vi "PC104_interface.vi"() -> ()   [LabVIEW 2016]
uses:
  Type_Defs/Digital_Out.ctl
  Type_Defs/Digital_In_1.ctl
  <vilib>/httpClient/ClientHandle.ctl
  Type_Defs/Analog_In.ctl
  msg7171_linux.llb/send single message.vi
  msg7171_linux.llb/send multiple messages.vi
  <vilib>/httpClient/POSTBuffer.vi
  <vilib>/httpClient/LabVIEWHTTPClient.lvlib
panel:
  out "GetAIO json":string
  out "GetDIO json":string
  in  "Get AIO":bool=TRUE
  in  "IR Lamps DutyCycle":dbl[][](array[numeric])
  in  "LN2 Platen":u16(slide) max=4095 step=1 scale=0.0..4095.0
  in  "LN2 Shroud":u16(slide) max=4095 step=1 scale=0.0..4095.0
  out "Digi_In_1":T1
  in  "Digi_Out":T2
  in  "Get DIO":bool=TRUE
  in  "exit":bool
  # "1"
  # "15"
  # "2"
  # "16"
  # "2               4                6                8                10              12              14              16"
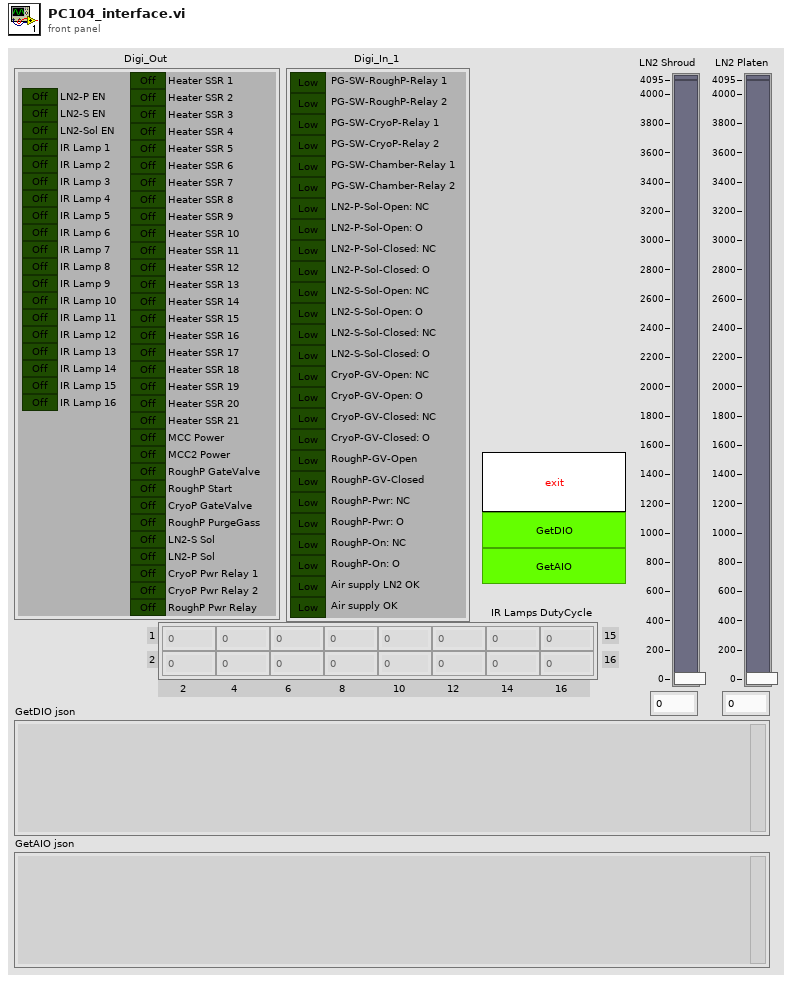
[diagram p1: front panel]
types:
  T1 = typedef "Digital_In_1.ctl" = cluster{"PG-SW-RoughP-Relay 1":bool, "PG-SW-RoughP-Relay 2":bool, "PG-SW-CryoP-Relay 1":bool, "PG-SW-CryoP-Relay 2":bool, "PG-SW-Chamber-Relay 1":bool, "PG-SW-Chamber-Relay 2":bool, "LN2-P-Sol-Open: NC":bool, "LN2-P-Sol-Open: O":bool, "LN2-P-Sol-Closed: NC":bool, "LN2-P-Sol-Closed: O":bool, "LN2-S-Sol-Open: NC":bool, "LN2-S-Sol-Open: O":bool, "LN2-S-Sol-Closed: NC":bool, "LN2-S-Sol-Closed: O":bool, "CryoP-GV-Open: NC":bool, "CryoP-GV-Open: O":bool, "CryoP-GV-Closed: NC":bool, "CryoP-GV-Closed: O":bool, "RoughP-GV-Open":bool, "RoughP-GV-Closed":bool, "RoughP-Pwr: NC":bool, "RoughP-Pwr: O":bool, "RoughP-On: NC":bool, "RoughP-On: O":bool, "Air supply LN2 OK":bool, "Air supply OK":bool}
  T2 = typedef "Digital_Out.ctl" = cluster{"LN2-P EN":bool, "LN2-S EN":bool, "LN2-Sol EN":bool, "IR Lamp 1":bool, "IR Lamp 2":bool, "IR Lamp 3":bool, "IR Lamp 4":bool, "IR Lamp 5":bool, "IR Lamp 6":bool, "IR Lamp 7":bool, "IR Lamp 8":bool, "IR Lamp 9":bool, "IR Lamp 10":bool, "IR Lamp 11":bool, "IR Lamp 12":bool, "IR Lamp 13":bool, "IR Lamp 14":bool, "IR Lamp 15":bool, "IR Lamp 16":bool, "Heater SSR 1":bool, "Heater SSR 2":bool, "Heater SSR 3":bool, "Heater SSR 4":bool, "Heater SSR 5":bool, "Heater SSR 6":bool, "Heater SSR 7":bool, "Heater SSR 8":bool, "Heater SSR 9":bool, "Heater SSR 10":bool, "Heater SSR 11":bool, "Heater SSR 12":bool, "Heater SSR 13":bool, "Heater SSR 14":bool, "Heater SSR 15":bool, "Heater SSR 16":bool, "Heater SSR 17":bool, "Heater SSR 18":bool, "Heater SSR 19":bool, "Heater SSR 20":bool, "Heater SSR 21":bool, "MCC Power":bool, "MCC2 Power":bool, "RoughP GateValve":bool, "RoughP Start":bool, "CryoP GateValve":bool, "RoughP PurgeGass":bool, "LN2-S Sol":bool, "LN2-P Sol":bool, "CryoP Pwr Relay 1":bool, "CryoP Pwr Relay 2":bool, "RoughP Pwr Relay":bool}
  T3 = typedef "LabVIEWHTTPClient.lvlib/ClientHandle.ctl" = refnum<k1>
  T4 = cluster{"go":bool, "Http session":T3, "URL prefex":string}
  T5 = typedef "Analog_In.ctl" = cluster{"Cabinet Temp 1":u16, "Cabinet Temp 2":u16, "Cabinet Temp 3":u16, "fs Front Door 1":u16, "fs Front Door 2":u16, "fs Front Door 3":u16, "fs Back Door 1":u16, "fs Back Door 2":u16, "fs Back Door 3":u16, "Rough Pump Temp":u16, "pg Chamber":u16, "pg Cryo Pump":u16, "pg Rough Pump":u16, "LN2 platen":u16, "LN2 shroud":u16}
  T6 = cluster{"out":cluster{"LN2 Platen":u16, "LN2 Shroud":u16}, "in":T5}
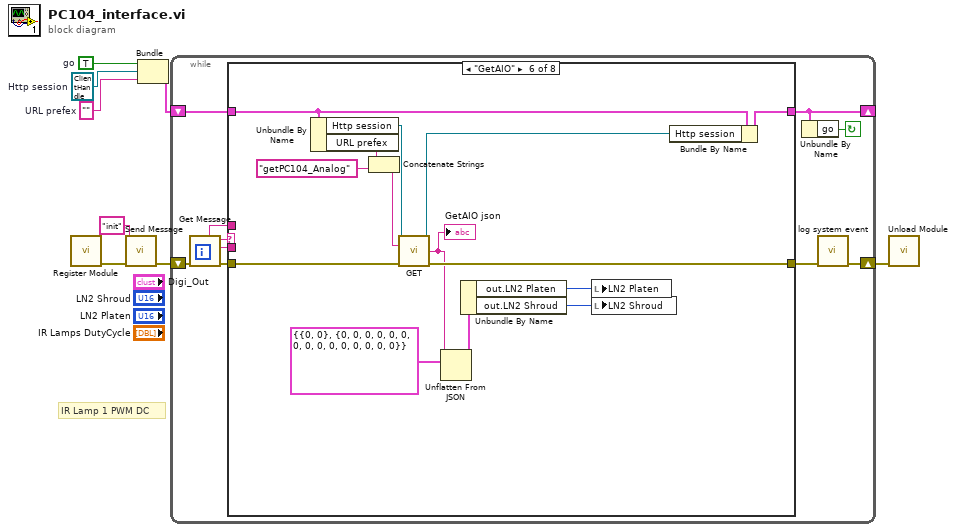
[diagram p0: block diagram]
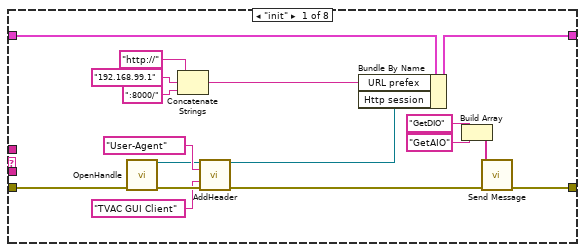
[diagram p2: hidden frame]
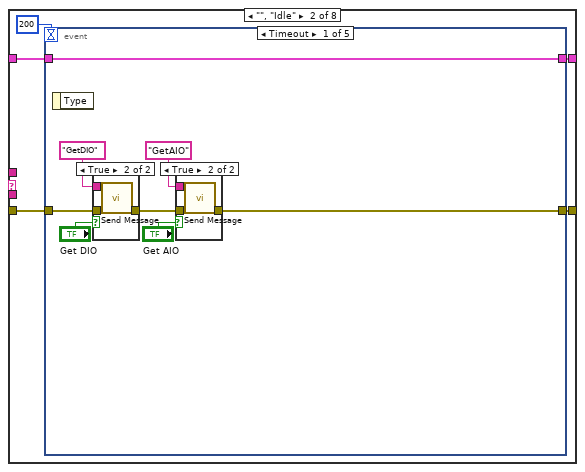
[diagram p3: hidden frame]
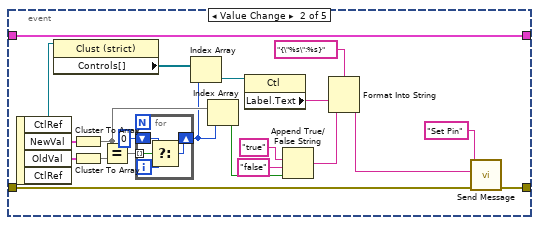
[diagram p6: hidden frame]
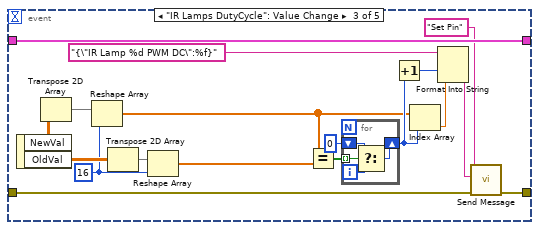
[diagram p7: hidden frame]
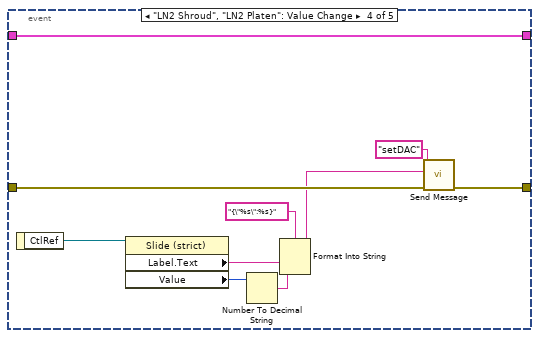
[diagram p8: hidden frame]
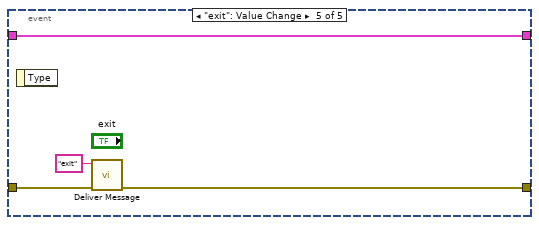
[diagram p9: hidden frame]
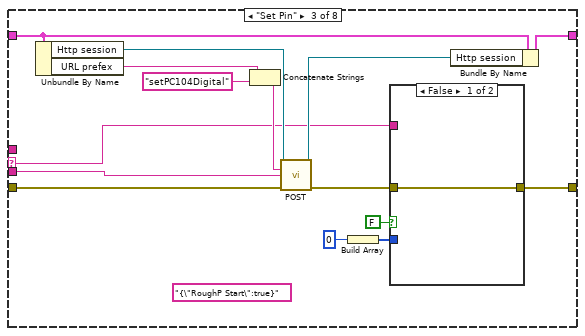
[diagram p10: hidden frame]
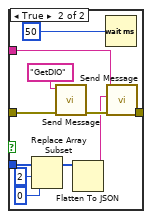
[diagram p11: hidden frame]
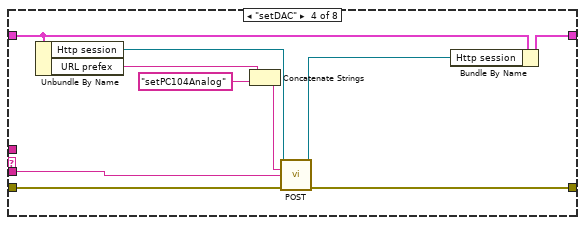
[diagram p12: hidden frame]
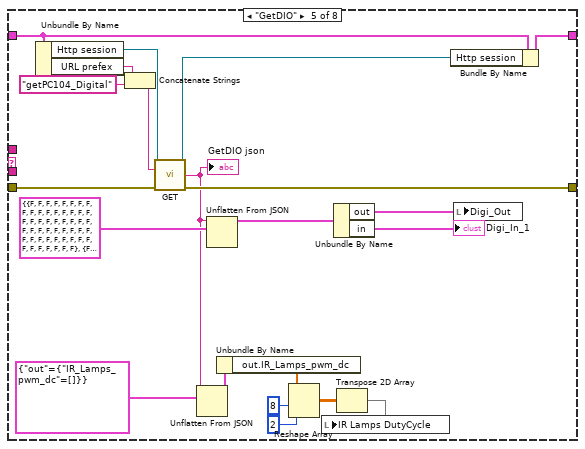
[diagram p13: hidden frame]
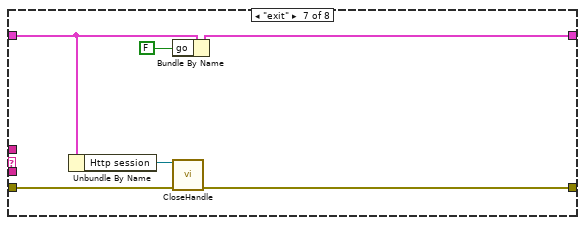
[diagram p14: hidden frame]
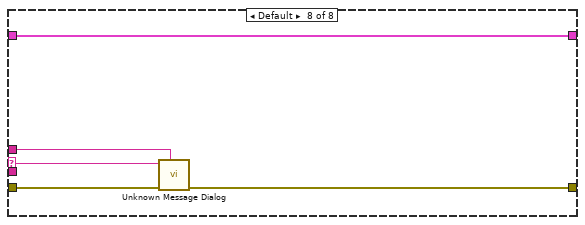
[diagram p15: hidden frame]
diagram:
  w4 = ""  # URL prefex
  w5 = T3 refnum  # Http session
  w6 = TRUE  # go
  # "IR Lamp 1 PWM DC"
  n1 = call "Register Module.vi"() -> ("error out"=w2:errorcluster)  [unwired: 10 in, 1 out]
  n2 = call-poly "Send Message.vi"("error in (no error)"=w2, "event"="init") -> ("error out"=w1:errorcluster)  [unwired: 9 in]
  n3 = Bundle("go"=w6, "Http session"=w5, "URL prefex"=w4) -> (w8:T4)  [unwired: 1 in]
  n4 = while {
    shift-left: w8 -> [w15]
    shift-right: [w12] -> _
    shift-right: [w10] -> w7
    shift-left: w1 -> [w18]
    stop <- w11 continue-if-true
    n5 = call "Get Message.vi"("error in (no error)"=w18) -> ("error out"=w16:errorcluster, "event buffer"=w17:string, "event"=w14:string, "source"=w13:string)  [unwired: 7 in]
    n6 = case shown="\"GetAIO\"" w14 {
      selector: w14 -> [_ _ w123 _ _ _ _ w198]
      tunnel: [w26 w37 w127 w149 w168 w182 w195 w200] -> w12
      tunnel: w15 -> [w35 w36 w126 w148 w167 w181 w190 w200]
      tunnel: w17 -> [_ _ w121 w145 _ _ _ _]
      tunnel: w16 -> [w30 w38 w125 w147 w170 w184 w193 w199]
      tunnel: w13 -> [_ _ _ _ _ _ _ w197]
      tunnel: [w22 w40 w124 w146 w169 w183 w192 w196] -> w9
      frame "init" {
        n7 = call <vilib>:"OpenHandle.vi"("error in (no error)"=w30) -> ("client handle out"=w31:T3, "error out"=w34:errorcluster)  [unwired: 13 in]
        n8 = Concatenate Strings("http://" ("url"), "192.168.99.1" ("Address"), ":8000/" ("url")) -> (w25:string)
        n9 = call <vilib>:"AddHeader.vi"("client handle"=w31, "header"="User-Agent", "value"="TVAC GUI Client", "error in (no error)"=w34) -> ("client handle out"=w24:T3, "error out"=w23:errorcluster)  [unwired: 10 in]
        n10 = Bundle By Name(cluster=w35, "URL prefex"=w25, "Http session"=w24) -> (w26:T4)
        n11 = Build Array("GetDIO" ("event"), "GetAIO" ("event")) -> (w20:string[])
        n12 = call-poly "Send Message.vi"("error in (no error)"=w23, "event"=w20) -> ("error out"=w22:errorcluster)  [unwired: 9 in]
      }
      frame "", "Idle" {
        n13 = event shown="[0] Timeout" {
          selector: _ -> [_ _ _ _ _]
          dyn-events: _ -> [_ _ _ _ _]
          timeout: 200 ("milliseconds to wait") -> [_ _ _ _ _]
          tunnel: w38 -> [w47 w72 w96 w111 w117]
          tunnel: [w42 w71 w95 w112 w116] -> w40
          tunnel: [w48 w77 w99 w104 w114] -> w37
          tunnel: w36 -> [w48 w77 w99 w104 w114]
          event Timeout {
            n14 = event-data() -> ()  [unwired: 1 in, 1 out]
            n15 = case shown="True" "Get DIO" {
              tunnel: w47 -> [w53 w56]
              tunnel: [w53 w55] -> w45
              tunnel: "GetDIO" ("event") -> [_ w54]
              frame False {
              }
              frame True {
                n16 = call-poly "Send Message.vi"("error in (no error)"=w56, "event"=w54) -> ("error out"=w55:errorcluster)  [unwired: 9 in]
              }
            }
            n17 = case shown="True" "Get AIO" {
              tunnel: w45 -> [w49 w52]
              tunnel: [w49 w51] -> w42
              tunnel: "GetAIO" ("event") -> [_ w50]
              frame False {
              }
              frame True {
                n18 = call-poly "Send Message.vi"("error in (no error)"=w52, "event"=w50) -> ("error out"=w51:errorcluster)  [unwired: 9 in]
              }
            }
          }
          event Value Change {
            n19 = event-data() -> ("CtlRef"=w58:refnum<vi>, "NewVal"=w73:T2, "OldVal"=w76:T2)  [unwired: 1 in, 1 out]
            n20 = property class="Clust (strict)"(reference=w58) -> ("Controls[]"=w68:refnum<vi>[])  [unwired: 1 in, 2 out]
            n21 = Cluster To Array(cluster=w73) -> (array=w69:bool[])
            n22 = Cluster To Array(cluster=w76) -> (array=w70:bool[])
            n23 = Equal?(x=w69, y=w70) -> (x = y?=w75:bool[])
            n24 = for {
              tunnel: w75 -> [w81] mode=indexing
              shift-right: [w80] -> w67
              shift-left: 0 -> [w79]
              i -> [w78]
              n25 = Select(t=w79, s=w81, f=w78) -> (s? t:f=w80:i32)
            }
            n26 = Index Array(array=w68, index=w67) -> (element=w66:refnum<vi>)
            n27 = Index Array(array=w69, index=w67) -> (element=w64:bool)
            n28 = property class="Ctl"(reference=w66) -> ("Label.Text"=w61:string)  [unwired: 1 in, 2 out]
            n29 = Append True/False String(1:w64, 2:"false" ("false string"), 3:"true" ("true string")) -> (0:w59:string)  [unwired: 1 in]
            n30 = Format Into String(format string="{\"%s\":%s}" ("string"), w61, w59) -> (resulting string=w57:string)  [unwired: 2 in, 1 out]
            n31 = call-poly "Send Message.vi"("error in (no error)"=w72, "event buffer"=w57, "event"="Set Pin") -> ("error out"=w71:errorcluster)  [unwired: 8 in]
          }
          event "IR Lamps DutyCycle": Value Change {
            w84 = 16 ("dimension size")
            n32 = event-data() -> ("NewVal"=w89:dbl[][], "OldVal"=w86:dbl[][])  [unwired: 1 in]
            n33 = Transpose 2D Array(2D array=w89) -> (transposed array=w90:dbl[][])
            n34 = Reshape Array(w90, w84) -> (w88:dbl[])
            n35 = Transpose 2D Array(2D array=w86) -> (transposed array=w87:dbl[][])
            n36 = Reshape Array(w87, w84) -> (w85:dbl[])
            n37 = Equal?(x=w88, y=w85) -> (x = y?=w98:bool[])
            n38 = for {
              tunnel: w98 -> [w103] mode=indexing
              shift-right: [w102] -> w91
              shift-left: 0 -> [w101]
              i -> [w100]
              n39 = Select(t=w101, s=w103, f=w100) -> (s? t:f=w102:i32)
            }
            n40 = Increment(x=w91) -> (x+1=w82:i32)
            n41 = Index Array(array=w88, index=w91) -> (element=w83:dbl)
            n42 = Format Into String(format string="{\"IR Lamp %d PWM DC\":%f}" ("string"), w82, w83) -> (resulting string=w92:string)  [unwired: 2 in, 1 out]
            n43 = call-poly "Send Message.vi"("error in (no error)"=w96, "event buffer"=w92, "event"="Set Pin") -> ("error out"=w95:errorcluster)  [unwired: 8 in]
          }
          event "LN2 Shroud", "LN2 Platen": Value Change {
            n44 = event-data() -> ("CtlRef"=w110:refnum<vi>)  [unwired: 1 in]
            n45 = property class="Slide (strict)"(reference=w110) -> ("Label.Text"=w108:string, "Value"=w107:u16)  [unwired: 1 in, 2 out]
            n46 = Number To Decimal String(number=w107) -> (decimal integer string=w106:string)  [unwired: 1 in]
            n47 = Format Into String(format string="{\"%s\":%s}" ("string"), w108, w106) -> (resulting string=w105:string)  [unwired: 2 in, 1 out]
            n48 = call-poly "Send Message.vi"("error in (no error)"=w111, "event buffer"=w105, "event"="setDAC") -> ("error out"=w112:errorcluster)  [unwired: 8 in]
          }
          event "exit": Value Change {
            n49 = event-data() -> ()  [unwired: 1 in, 1 out]
            n50 = call "Deliver Message.vi"("error in (no error)"=w117, "event"="exit") -> ("error out"=w116:errorcluster)  [unwired: 9 in]
          }
        }
      }
      frame "Set Pin" {
        (unwired) "{\"RoughP Start\":true}" ("string")
        n51 = Unbundle By Name(w126) -> ("Http session"=w131:T3, "URL prefex"=w129:string)
        n52 = Concatenate Strings(w129, "setPC104Digital" ("url")) -> (w130:string)
        n53 = call-poly <vilib>:"POST.vi"("client handle"=w131, "url"=w130, "buffer"=w121, "error in (no error)"=w125) -> ("client handle out"=w132:T3, "error out"=w122:errorcluster)  [unwired: 8 in, 2 out]
        n54 = Build Array(0) -> (w119:i32[])
        n55 = case shown="False" FALSE {
          tunnel: [w133 w144] -> w124
          tunnel: w123 -> [_ w143]
          tunnel: w122 -> [w133 w142]
          tunnel: w119 -> [_ w139]
          frame False {
          }
          frame True {
            n56 = Replace Array Subset(array=w139, new element=0 ("new element/subarray"), index=2) -> (w135:i32[])
            n57 = call-poly "Send Message.vi"("error in (no error)"=w142, "event"="GetDIO") -> ("error out"=w141:errorcluster)  [unwired: 9 in]
            n58 = Flatten To JSON(anything=w135) -> (JSON string=w136:string)  [unwired: 2 in, 1 out]
            n59 = Wait (ms)(milliseconds to wait=u32 50) -> ()  [unwired: 1 out]
            n60 = call-poly "Send Message.vi"("error in (no error)"=w141, "event buffer"=w136, "event"=w143) -> ("error out"=w144:errorcluster)  [unwired: 8 in]
          }
        }
        n61 = Bundle By Name(cluster=w126, "Http session"=w132) -> (w127:T4)
      }
      frame "setDAC" {
        n62 = Unbundle By Name(w148) -> ("Http session"=w153:T3, "URL prefex"=w151:string)
        n63 = Concatenate Strings(w151, "setPC104Analog" ("url")) -> (w152:string)
        n64 = call-poly <vilib>:"POST.vi"("client handle"=w153, "url"=w152, "buffer"=w145, "error in (no error)"=w147) -> ("client handle out"=w154:T3, "error out"=w146:errorcluster)  [unwired: 8 in, 2 out]
        n65 = Bundle By Name(cluster=w148, "Http session"=w154) -> (w149:T4)
      }
      frame "GetDIO" {
        n66 = Unbundle By Name(w167) -> ("Http session"=w174:T3, "URL prefex"=w172:string)
        n67 = Concatenate Strings(w172, "getPC104_Digital" ("url")) -> (w173:string)
        n68 = call <vilib>:"GET.vi"("client handle"=w174, "url"=w173, "error in (no error)"=w170) -> ("client handle out"=w175:T3, "body"=w155:string, "error out"=w169:errorcluster)  [unwired: 9 in, 1 out]
        "GetDIO json" <- w155
        n69 = Unflatten From JSON(JSON string=w155, type and defaults=cluster{"out":cluster{"IR_Lamps_pwm_dc":dbl[]}} {"out"={"IR_Lamps_pwm_dc"=[]}}) -> (value=w157:cluster{"out":cluster{"IR_Lamps_pwm_dc":dbl[]}})  [unwired: 5 in, 1 out]
        n70 = Unflatten From JSON(JSON string=w155, type and defaults=cluster{"out":T2, "in":T1} {"out"={"LN2-P EN"=FALSE, "LN2-S EN"=FALSE, "LN2-Sol EN"=FALSE, "IR Lamp 1"=FALSE, "IR Lamp 2"=FALSE, "IR Lamp 3"=FALSE, "IR Lamp 4"=FALSE, "IR Lamp 5"=FALSE, "IR Lamp 6"=FALSE, "IR Lamp 7"=FALSE, "IR Lamp 8"=FALSE, "IR Lamp 9"=FALSE, "IR Lamp 10"=FALSE, "IR Lamp 11"=FALSE, "IR Lamp 12"=FALSE, "IR Lamp 13"=FALSE, "IR Lamp 14"=FALSE, "IR Lamp 15"=FALSE, "IR Lamp 16"=FALSE, "Heater SSR 1"=FALSE, "Heater SSR 2"=FALSE, "Heater SSR 3"=FALSE, "Heater SSR 4"=FALSE, "Heater SSR 5"=FALSE, "Heater SSR 6"=FALSE, "Heater SSR 7"=FALSE, "Heater SSR 8"=FALSE, "Heater SSR 9"=FALSE, "Heater SSR 10"=FALSE, "Heater SSR 11"=FALSE, "Heater SSR 12"=FALSE, "Heater SSR 13"=FALSE, "Heater SSR 14"=FALSE, "Heater SSR 15"=FALSE, "Heater SSR 16"=FALSE, "Heater SSR 17"=FALSE, "Heater SSR 18"=FALSE, "Heater SSR 19"=FALSE, "Heater SSR 20"=FALSE, "Heater SSR 21"=FALSE, "MCC Power"=FALSE, "MCC2 Power"=FALSE, "RoughP GateValve"=FALSE, "RoughP Start"=FALSE, "CryoP GateValve"=FALSE, "RoughP PurgeGass"=FALSE, "LN2-S Sol"=FALSE, "LN2-P Sol"=FALSE, "CryoP Pwr Relay 1"=FALSE, "CryoP Pwr Relay 2"=FALSE, "RoughP Pwr Relay"=FALSE}, "in"={"PG-SW-RoughP-Relay 1"=FALSE, "PG-SW-RoughP-Relay 2"=FALSE, "PG-SW-CryoP-Relay 1"=FALSE, "PG-SW-CryoP-Relay 2"=FALSE, "PG-SW-Chamber-Relay 1"=FALSE, "PG-SW-Chamber-Relay 2"=FALSE, "LN2-P-Sol-Open: NC"=FALSE, "LN2-P-Sol-Open: O"=FALSE, "LN2-P-Sol-Closed: NC"=FALSE, "LN2-P-Sol-Closed: O"=FALSE, "LN2-S-Sol-Open: NC"=FALSE, "LN2-S-Sol-Open: O"=FALSE, "LN2-S-Sol-Closed: NC"=FALSE, "LN2-S-Sol-Closed: O"=FALSE, "CryoP-GV-Open: NC"=FALSE, "CryoP-GV-Open: O"=FALSE, "CryoP-GV-Closed: NC"=FALSE, "CryoP-GV-Closed: O"=FALSE, "RoughP-GV-Open"=FALSE, "RoughP-GV-Closed"=FALSE, "RoughP-Pwr: NC"=FALSE, "RoughP-Pwr: O"=FALSE, "RoughP-On: NC"=FALSE, "RoughP-On: O"=FALSE, "Air supply LN2 OK"=FALSE, "Air supply OK"=FALSE}}) -> (value=w163:cluster{"out":T2, "in":T1})  [unwired: 5 in, 1 out]
        n71 = Unbundle By Name(w157) -> ("out.IR_Lamps_pwm_dc"=w156:dbl[])
        n72 = Reshape Array(w156, 8 ("dimension size"), 2 ("dimension size")) -> (w160:dbl[][])
        n73 = Unbundle By Name(w163) -> ("out"=w166:T2, "in"=→"Digi_In_1":T1)
        n74 = Transpose 2D Array(2D array=w160) -> (transposed array=w159:dbl[][])
        n75 = local write "IR Lamps DutyCycle"(w159) -> ()
        n76 = Bundle By Name(cluster=w167, "Http session"=w175) -> (w168:T4)
        n77 = local write "Digi_Out"(w166) -> ()
      }
      frame "GetAIO" {
        n78 = Unbundle By Name(w181) -> ("Http session"=w188:T3, "URL prefex"=w186:string)
        n79 = Concatenate Strings(w186, "getPC104_Analog" ("url")) -> (w187:string)
        n80 = call <vilib>:"GET.vi"("client handle"=w188, "url"=w187, "error in (no error)"=w184) -> ("client handle out"=w189:T3, "body"=w176:string, "error out"=w183:errorcluster)  [unwired: 9 in, 1 out]
        "GetAIO json" <- w176
        n81 = Unflatten From JSON(JSON string=w176, type and defaults=T6 {"out"={"LN2 Platen"=0, "LN2 Shroud"=0}, "in"={"Cabinet Temp 1"=0, "Cabinet Temp 2"=0, "Cabinet Temp 3"=0, "fs Front Door 1"=0, "fs Front Door 2"=0, "fs Front Door 3"=0, "fs Back Door 1"=0, "fs Back Door 2"=0, "fs Back Door 3"=0, "Rough Pump Temp"=0, "pg Chamber"=0, "pg Cryo Pump"=0, "pg Rough Pump"=0, "LN2 platen"=0, "LN2 shroud"=0}}) -> (value=w179:T6)  [unwired: 5 in, 1 out]
        n82 = Unbundle By Name(w179) -> ("out.LN2 Platen"=w178:u16, "out.LN2 Shroud"=w177:u16)
        n83 = local write "LN2 Platen"(w178) -> ()
        n84 = local write "LN2 Shroud"(w177) -> ()
        n85 = Bundle By Name(cluster=w181, "Http session"=w189) -> (w182:T4)
      }
      frame "exit" {
        n86 = Unbundle By Name(w190) -> ("Http session"=w191:T3)
        n87 = Bundle By Name(cluster=w190, "go"=FALSE ("Bundle Element")) -> (w195:T4)
        n88 = call <vilib>:"CloseHandle.vi"("client handle"=w191, "error in (no error)"=w193) -> ("error out"=w192:errorcluster)  [unwired: 13 in]
      }
      frame Default {
        n89 = call "Unknown Message Dialog.vi"("source"=w197, "error in (no error)"=w199, "event name"=w198) -> ("error out"=w196:errorcluster)  [unwired: 8 in]
      }
    }
    n90 = Unbundle By Name(w12) -> ("go"=w11:bool)
    n91 = call "log system event.vi"("error in (no error)"=w9) -> ("error out"=w10:errorcluster)  [unwired: 9 in, 1 out]
  }
  n92 = call "Unload Module.vi"("error in (no error)"=w7) -> ()  [unwired: 10 in, 1 out]
